vi "Transmitter_RSMA - 3 SC - With timer.vi"() -> ()   [LabVIEW 2022 SP3]
uses:
  <instrlib>/niUSRP/niUSRP Write Tx Data (CDB).vi
panel:
  in  "Iterations":i32=10000
  out "Time(s)":sgl format="%#_4g"
  in  "Beta/Alpha":dbl(slide)=0.17500000000000002 step=0.005 scale=0.0..1.0
  in  "Alpha":dbl(slide)=0.49999999999999994 step=0.005 scale=0.0..1.0
  in  "Tab Control":enum32{"USRP Parameters", "Transmission"}(tab)
  in  "USRP ControledParameters 2":T1={"Active Antenna"="TX1", "Gain (dB)"=0.0, "Carrier Frequency"=2400000000.0, "IQ Rate"=2000000.0, "Active Channel"="0"} {"IQ Rate" format="%#_6p"; "Carrier Frequency" format="%#_6p"; "Gain (dB)" format="%#_6f"}
  in  "Device selection":refnum<k15>="RIO0"
  in  "stop":bool
  out "Error out":errorcluster
  in  "Modulation parameter":T2
  out "Bits length":i32
  out "Bits length 2":i32
  out "Frame Duration":dbl format="%#_6p"
  out "Coerced Parameters":T3={"IQ Rate"=100000.0, "Carrier  Freq."=100000.0, "Gain"=0.0} {"Gain" format="%#_6f"; "Carrier  Freq." format="%#_6p"; "IQ Rate" format="%#_6p"}
  out "Transmitted Waveform":dbl[](graph)
  in  "Message 2":string="ptua. At vero eos et accusam et justo duo dolores et ea rebum. Stet clita kasd gubergren, no sea takimata sanctus est Lorem ipsum dolor sit amet. Lore"
  in  "Message 1":string="Lorem ipsum dolor sit amet, consetetur sadipscing elitr, sed diam nonumy eirmod tempor invidunt ut labore et dolore magna aliquyam erat, sed diam volu"
  in  "error in (no error)":errorcluster
  # "RSMA Transmitter"
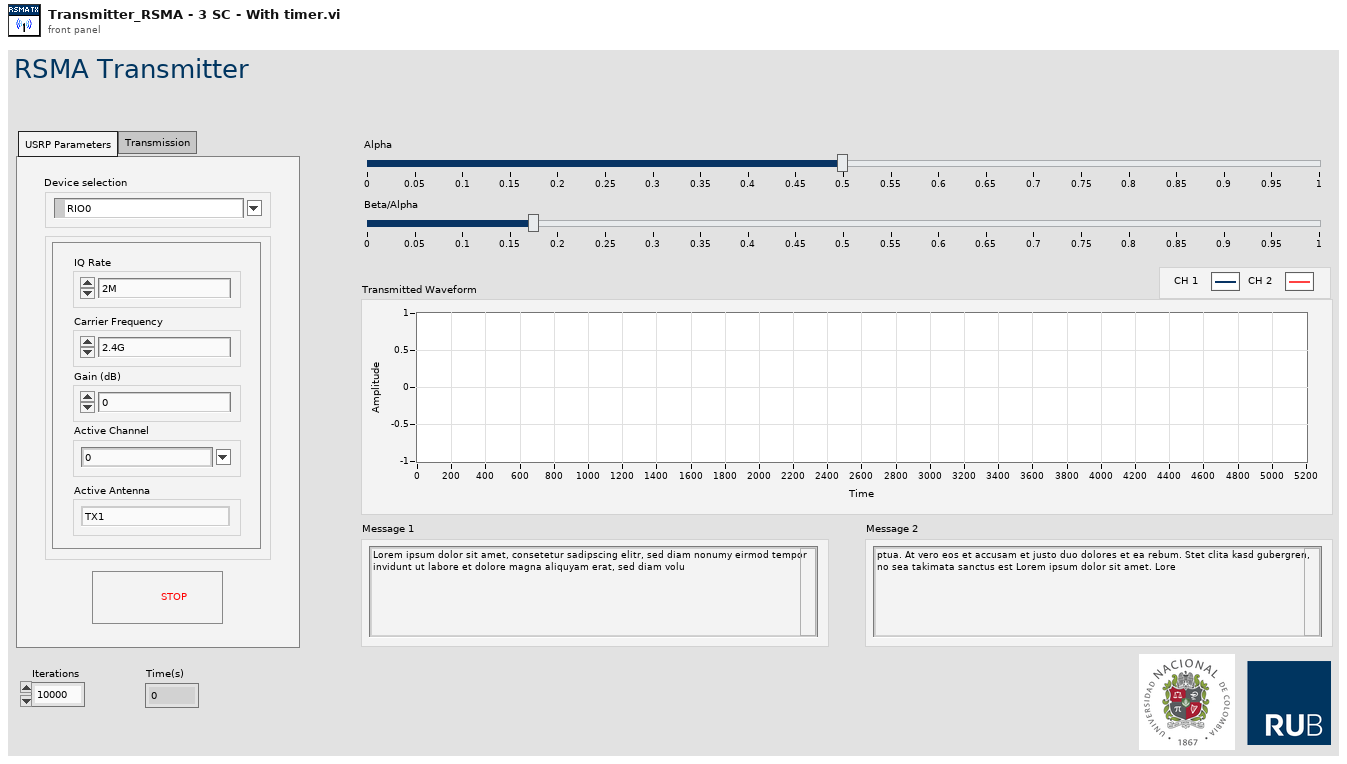
[diagram p1: front panel]
types:
  T1 = cluster{"Active Antenna":string, "Gain (dB)":dbl, "Carrier Frequency":dbl, "IQ Rate":dbl, "Active Channel":string}
  T2 = cluster{"Modulation type":enum16{"QPSK(4QAM)", "64QAM", "16QAM", "BPSK"}, "BCC rate (k/n)":enum16{"1/2", "2/3", "3/4"}}
  T3 = cluster{"IQ Rate":dbl, "Carrier  Freq.":dbl, "Gain":dbl}
  T4 = cluster{"coerced IQ rate":dbl, "coerced carrier frequency":dbl, "coerced gain":dbl}
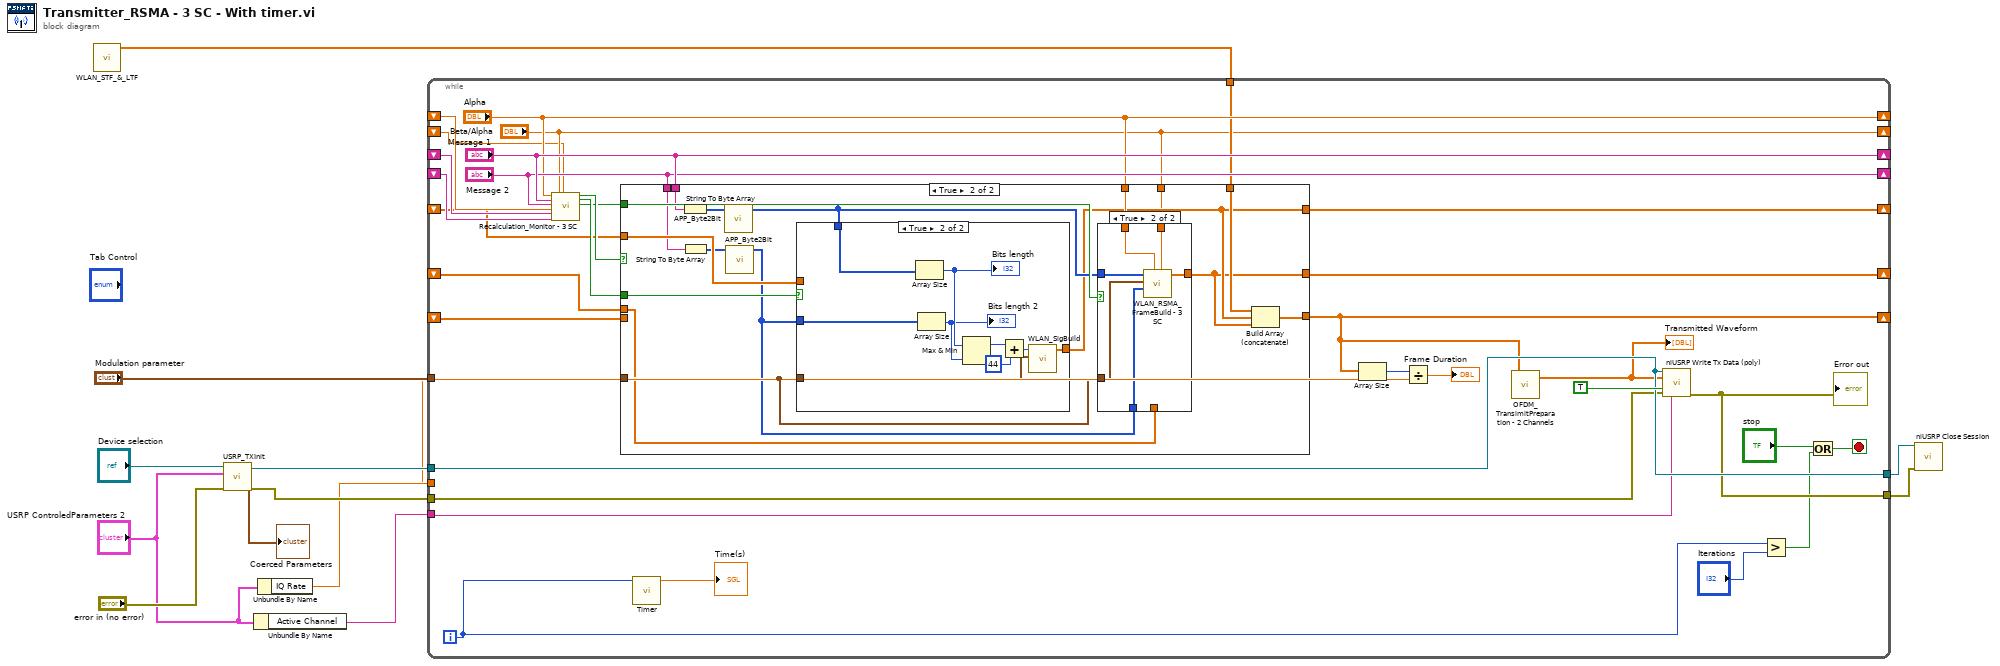
[diagram p0: block diagram]
diagram:
  n1 = call "WLAN_STF_&_LTF.vi"() -> ("STF & LTF"=w1:cdb[])  [unwired: 11 in]
  n2 = call "USRP_TXInit.vi"("device names"="Device selection", "USRP ControledParameters"="USRP ControledParameters 2", "error in (no error)"="error in (no error)") -> ("session handle out"=w11:refnum<k15>, "USRP CoercedParamters"=→"Coerced Parameters":T4, "error out"=w10:errorcluster)  [unwired: 5 in]
  n3 = Unbundle By Name("USRP ControledParameters 2") -> ("Active Channel"=w3:string)
  n4 = Unbundle By Name("USRP ControledParameters 2") -> ("IQ Rate"=w9:dbl)
  n5 = while {
    tunnel: w11 -> [w43]
    tunnel: w10 -> [w23]
    tunnel: w9 -> [w42]
    tunnel: [w43] -> w8
    tunnel: [w41] -> w7
    tunnel: w3 -> [w40]
    shift-right: ["Alpha"] -> _
    shift-left: _ -> [w39]
    shift-right: ["Message 1"] -> _
    shift-left: _ -> [w38]
    shift-right: ["Message 2"] -> _
    shift-left: _ -> [w37]
    tunnel: "Modulation parameter" -> [w31]
    shift-right: [w30] -> _
    shift-left: _ -> [w29]
    shift-right: [w27] -> _
    shift-left: _ -> [w26]
    tunnel: w1 -> [w25]
    shift-right: [w22] -> _
    shift-left: _ -> [w24]
    shift-right: ["Beta/Alpha"] -> _
    shift-left: _ -> [w19]
    i -> [w14]
    stop <- w16 stop-if-true
    n6 = call "Recalculation_Monitor - 3 SC.vi"("Alpha"="Alpha", "Message 1"="Message 1", "Message 2"="Message 2", "Alpha old"=w39, "Message 1 old"=w38, "Message 2 old"=w37, "Beta/Alpha"="Beta/Alpha", "Beta/Alpha old"=w19) -> ("Recalculate?"=w36:bool, "Recalculate SIG"=w35:bool, "Recalculate OFDM"=w34:bool)  [unwired: 9 in]
    n7 = case shown="True" w36 {
      tunnel: w35 -> [_ w66]
      tunnel: w34 -> [_ w65]
      tunnel: "Message 1" -> [_ w60]
      tunnel: "Message 2" -> [_ w61]
      tunnel: w31 -> [_ w57]
      tunnel: [w49 w53] -> w30
      tunnel: w29 -> [w49 w64]
      tunnel: "Alpha" -> [_ w56]
      tunnel: [w48 w52] -> w27
      tunnel: w26 -> [w48 w55]
      tunnel: w25 -> [_ w54]
      tunnel: [w47 w51] -> w22
      tunnel: w24 -> [w47 _]
      tunnel: "Beta/Alpha" -> [_ w50]
      frame False {
      }
      frame True {
        n8 = String To Byte Array(string=w60) -> (unsigned byte array=w62:u8[])
        n9 = String To Byte Array(string=w61) -> (unsigned byte array=w63:u8[])
        n10 = call "APP_Byte2Bit.vi"("input byte stream"=w62) -> ("output bit stream"=w58:i8[])  [unwired: 10 in]
        n11 = call "APP_Byte2Bit.vi"("input byte stream"=w63) -> ("output bit stream"=w59:i8[])  [unwired: 10 in]
        n12 = case shown="True" w66 {
          tunnel: w57 -> [_ w75]
          tunnel: [w74 w81] -> w53
          tunnel: w64 -> [w74 _]
          tunnel: w59 -> [_ w77]
          tunnel: w58 -> [_ w76]
          frame False {
          }
          frame True {
            n13 = Array Size(array=w76) -> (size(s)=w83:i32)
            "Bits length" <- w83
            n14 = Array Size(array=w77) -> (size(s)=w82:i32)
            "Bits length 2" <- w82
            n15 = Max & Min(x=w83, y=w82) -> (max(x,y)=w79:i32)  [unwired: 1 out]
            n16 = Add(x=w79, y=44) -> (x+y=w80:i32)
            n17 = call "WLAN_SigBuild.vi"("Data bit length"=w80, "Modulation parameter"=w75) -> ("symbols"=w81:cdb[])  [unwired: 7 in, 1 out]
          }
        }
        n18 = case shown="True" w65 {
          tunnel: w59 -> [_ w73]
          tunnel: w58 -> [_ w72]
          tunnel: w57 -> [_ w71]
          tunnel: w56 -> [_ w70]
          tunnel: [w67 w69] -> w52
          tunnel: w55 -> [w67 _]
          tunnel: w50 -> [_ w68]
          frame False {
          }
          frame True {
            n19 = call "WLAN_RSMA_FrameBuild - 3 SC.vi"("Beta/Alpha"=w68, "Alpha"=w70, "data in 2"=w73, "Modulation parameter"=w71, "data in"=w72) -> ("output array"=w69:cdb[])  [unwired: 5 in, 1 out]
          }
        }
        n20 = Build Array (concatenate)(w54, w53, w52) -> (w51:cdb[])
      }
    }
    n21 = call "Timer.vi"("index"=w14) -> ("Time(s)"=→"Time(s)":sgl)  [unwired: 10 in]
    n22 = Array Size(array=w22) -> (size(s)=w45:i32)
    n23 = Divide(x=w45, y=w42) -> (x/y=→"Frame Duration":dbl)
    n24 = call "OFDM_TransimitPreparation - 2 Channels.vi"("array"=w22) -> ("output array"=w21:cdb[])  [unwired: 8 in, 2 out]
    "Transmitted Waveform" <- w21
    n25 = call-poly <instrlib>:"niUSRP Write Tx Data (poly).vi"("session handle"=w43, "channel list"=w40, "data"=w21, "end of data?"=TRUE, "error in (no error)"=w23) -> ("error out"=w41:errorcluster)  [unwired: 9 in, 1 out]
    "Error out" <- w41
    n26 = Greater?(x=w14, y="Iterations") -> (0:w15:bool)
    n27 = Or(x="stop", y=w15) -> (x .or. y?=w16:bool)
  }
  n28 = call <instrlib>:"niUSRP Close Session.vi"("session handle"=w8, "error in (no error)"=w7) -> ()  [unwired: 13 in, 1 out]
